vi "initMessages.vi"(7 "GainsCluster":T1, 8 "error in (no error)":errorcluster, 9 "Argument Setpoint":dbl, 10 "Modulus Setpoint":dbl, 11 "writer name in":refnum<k21>) -> (0 "error out":errorcluster, 3 "Refnum out":refnum<k21>)   [LabVIEW 2012]
uses:
  Messages.ctl
  messageTypes.ctl
  GainsTDef.ctl
  setpointCluster.ctl
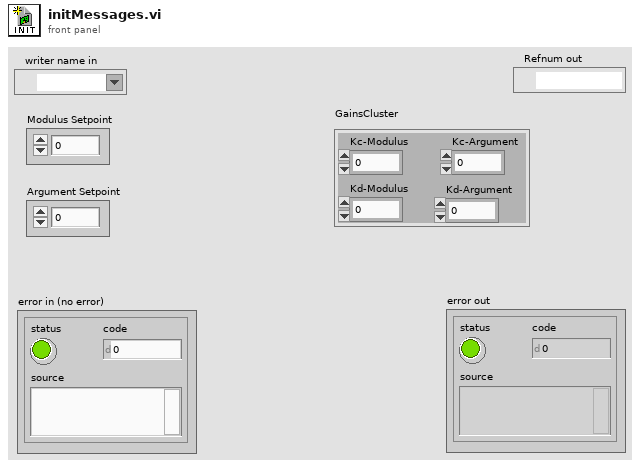
[diagram p1: front panel]
types:
  T1 = typedef "GainsTDef.ctl" = cluster{"Kc-Modulus":dbl, "Kd-Modulus":dbl, "Kc-Argument":dbl, "Kd-Argument":dbl}
  T2 = typedef "Messages.ctl" = cluster{"message data":variant, "message type":T3}
  T3 = typedef "messageTypes.ctl" = enum16{"Speeds", "Stop", "PolarCoordinates", "Gains", "Setpoints"}
  T4 = typedef "setpointCluster.ctl" = cluster{"Modulus Setpoint":dbl, "Argument Setpoint":dbl}
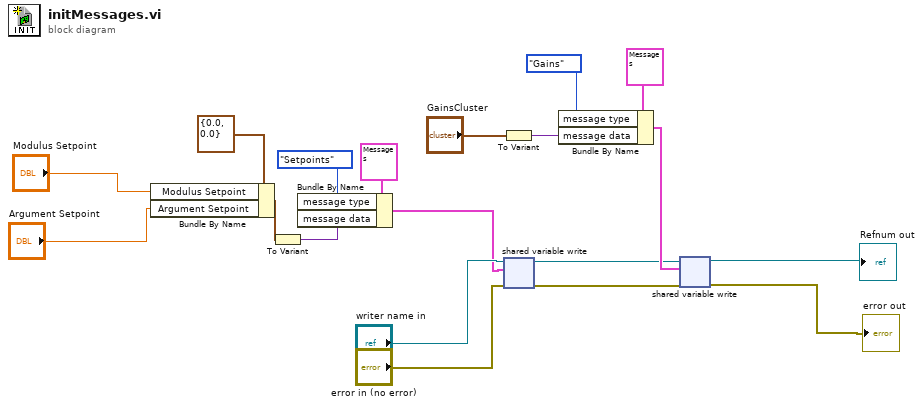
[diagram p0: block diagram]
diagram:
  n1 = Bundle By Name(cluster=T4 {"Modulus Setpoint"=0.0, "Argument Setpoint"=0.0} ("Setpoint Cluster"), "Modulus Setpoint"="Modulus Setpoint", "Argument Setpoint"="Argument Setpoint") -> (w14:T4)
  n2 = To Variant(anything=w14) -> (Variant=w13:variant)
  n3 = Bundle By Name(cluster=T2 {"message data"=variant, "message type"=enum."Stop"} ("message"), "message type"=messageTypes."Setpoints", "message data"=w13) -> (w17:T2)
  n4 = To Variant(anything="GainsCluster") -> (Variant=w7:variant)
  n5 = shared-variable-write("writer name in", "error in (no error)", w17) -> (w4:refnum<k21>, w3:errorcluster)  [unwired: 1 in, 1 out]
  n6 = Bundle By Name(cluster=T2 {"message data"=variant, "message type"=enum."Stop"} ("message"), "message type"=messageTypes."Gains", "message data"=w7) -> (w5:T2)
  n7 = shared-variable-write(w4, w3, w5) -> (→"Refnum out":refnum<k21>, →"error out":errorcluster)  [unwired: 1 in, 1 out]
